vi "WS1021 demo GUI settings.vi"(9 "Demo Mode":enum32{"Live mode", "Virtual mode"}(radio), 10 "VNA ports":bool[](array[boolean])=[TRUE, FALSE, FALSE, FALSE], 11 "Settings":T1={"Specification"={"States"=32, "Cmin"=250.0, "Cmax"=2600.0}, "Extraction frequencies"={"Frequency for C (MHz)"=900.0, "Frequency for Q (MHz)"=2000.0, "Frequency, C_DC (MHz)"=100.0}, "Timeout (ms)"=250, "Model"=enum."pi", "Topology"=enum."Series", "Error limits"=path ""}) -> (1 "Demo Mode out":enum32{"Live mode", "Virtual mode"}(radio), 2 "VNA ports out":bool[](array[boolean])=[TRUE, FALSE, FALSE, FALSE], 3 "Settings out":T1={"Specification"={"States"=32, "Cmin"=250.0, "Cmax"=2600.0}, "Extraction frequencies"={"Frequency for C (MHz)"=900.0, "Frequency for Q (MHz)"=2000.0, "Frequency, C_DC (MHz)"=100.0}, "Timeout (ms)"=250, "Model"=enum."pi", "Topology"=enum."Series", "Error limits"=path ""})   [LabVIEW 2020]
uses:
  WS1021 demo GUI settings.ctl
panel:
  in  "System Cancel Button":bool
  in  "System OK Button":bool
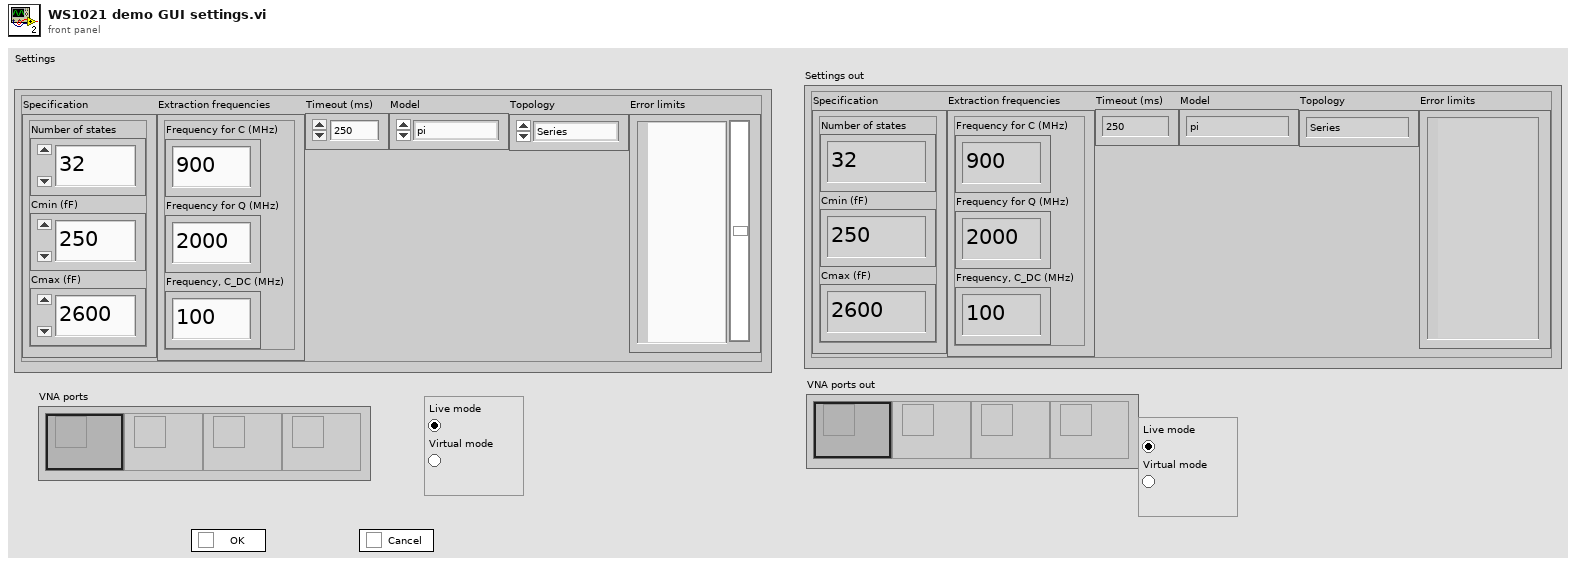
[diagram p1: front panel]
types:
  T1 = typedef "WS1021 demo GUI settings.ctl" = cluster{"Specification":cluster{"States":i32, "Cmin":dbl, "Cmax":dbl}, "Extraction frequencies":cluster{"Frequency for C (MHz)":dbl, "Frequency for Q (MHz)":dbl, "Frequency, C_DC (MHz)":dbl}, "Timeout (ms)":i32, "Model":enum16{"pi", "tee"}, "Topology":enum16{"Series", "Parallel"}, "Error limits":path}
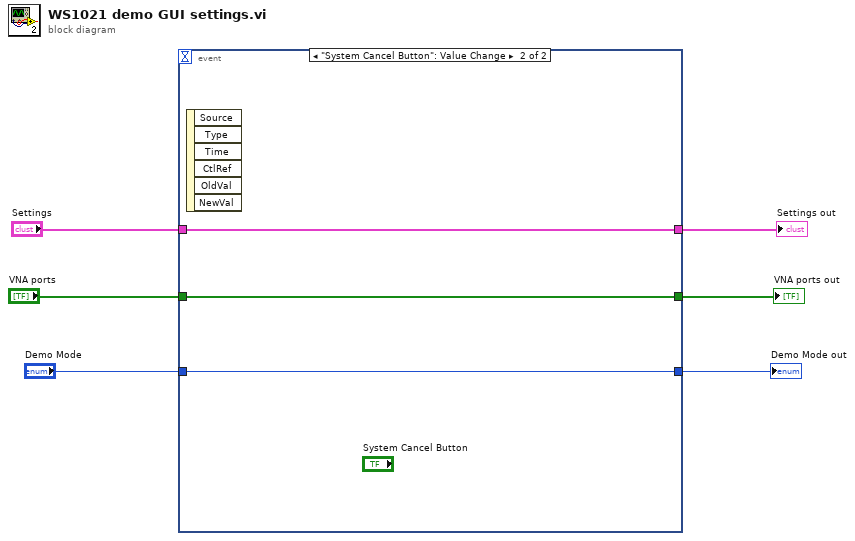
[diagram p0: block diagram]
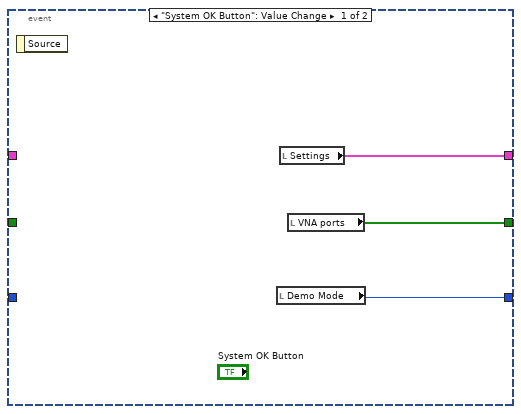
[diagram p2: hidden frame]
diagram:
  n1 = event shown="[1] \"System Cancel Button\": Value Change" {
    selector: _ -> [_ _]
    dyn-events: _ -> [_ _]
    timeout: _ -> [_ _]
    tunnel: "Settings" -> [_ w12]
    tunnel: "VNA ports" -> [_ w11]
    tunnel: [w8 w12] -> w3
    tunnel: [w9 w11] -> w4
    tunnel: [w7 w10] -> w2
    tunnel: "Demo Mode" -> [_ w10]
    event "System OK Button": Value Change {
      n2 = event-data() -> ()  [unwired: 1 in, 1 out]
      n3 = local read "Demo Mode"() -> (w7:enum32{"Live mode", "Virtual mode"})
      n4 = local read "Settings"() -> (w8:T1)
      n5 = local read "VNA ports"() -> (w9:bool[])
    }
    event "System Cancel Button": Value Change {
      n6 = event-data() -> ()  [unwired: 1 in, 6 out]
    }
  }
  "VNA ports out" <- w4
  "Settings out" <- w3
  "Demo Mode out" <- w2
